vi "Count true in array.vi"(11 "Wash Options":bool[](array[boolean])) -> (3 "Numeric":i32)   [LabVIEW 2024]
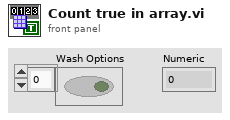
[diagram p1: front panel]
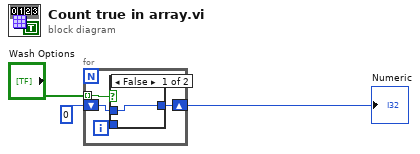
[diagram p0: block diagram]
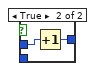
[diagram p2: hidden frame]
diagram:
  n1 = for {
    tunnel: "Wash Options" -> [w7] mode=indexing
    shift-right: [w5] -> w3
    shift-left: 0 -> [w4]
    i -> [w6]
    n2 = case shown="False" w7 {
      tunnel: w6 -> [_ _]
      tunnel: [w8 w10] -> w5
      tunnel: w4 -> [w8 w9]
      frame False {
      }
      frame True {
        n3 = Increment(x=w9) -> (x+1=w10:i32)
      }
    }
  }
  "Numeric" <- w3
